vi "FFTSemDC.vi"(2 "wfm":waveform(dbl), 6 "Fase":bool) -> (16 "FFT":cluster{"f0":dbl, "df":dbl, "magnitude":dbl[]})   [LabVIEW 2017]
uses:
  <vilib>/measure/madcrms.llb/Basic Averaged DC-RMS for 1 Chan.vi
  <vilib>/express/express analysis/Spectral/Block/exnSpectralBlock spectral measurements peak poly.vi
  <vilib>/express/express analysis/Spectral/Block/exnSpectralBlock spectral measurements peak WFM.vi
  <vilib>/express/express analysis/Spectral/XNode/ExpressSpectralMeasurementsBlockNode.xnode
  <vilib>/measure/NI_MAPro.lvlib
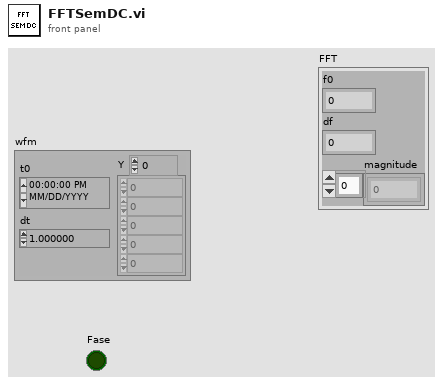
[diagram p1: front panel]
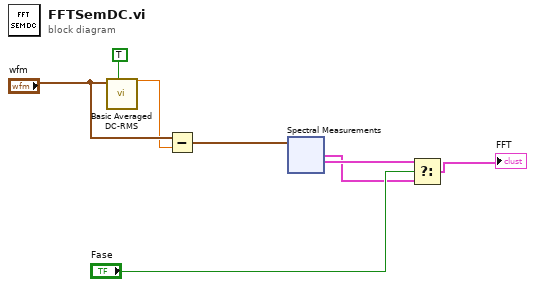
[diagram p0: block diagram]
diagram:
  n1 = call-poly <vilib>:"Basic Averaged DC-RMS.vi"("reset"=TRUE, "signal in"="wfm") -> ("DC value"=w6:dbl)  [unwired: 6 in, 3 out]
  n2 = Subtract(x="wfm", y=w6) -> (x-y=w1:waveform(dbl))
  n3 = xnode "Spectral Measurements"("Signals"=w1) -> ("FFT - (Peak)"=w3:cluster{"f0":dbl, "df":dbl, "magnitude":dbl[]}, "Phase"=w4:cluster{"f0":dbl, "df":dbl, "phase":dbl[]})  [unwired: 1 in, 1 out]
  n4 = Select(t=w4, s="Fase", f=w3) -> (s? t:f=→"FFT":cluster{"f0":dbl, "df":dbl, "magnitude":dbl[]})
